vi "Rising Edge Detector.vi"(11 "Input":bool) -> (3 "Rising edge?":bool)   [LabVIEW 2018]
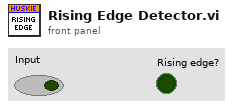
[diagram p1: front panel]
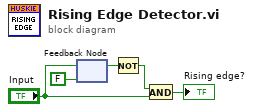
[diagram p0: block diagram]
diagram:
  n1 = feedback #1(FALSE ("Input")) -> (w5:bool)
  n2 = feedback-in #1("Input") -> ()
  n3 = Not(x=w5) -> (.not. x?=w1:bool)
  n4 = And(x=w1, y="Input") -> (x .and. y?=→"Rising edge?":bool)
